vi "Icon_Adapt Format Cluster for Storage.vi"(8 "Error":errorcluster, 11 "Colors":T1={"Header"="", "Format"={"Color"={"Body txt"=255, "Body Back"=12632256, "Frame"=0, "Header txt"=32768, "Header Back"=16744703, "type"=enum."2 Color"}, "Icon Sizing"={"Rule"=enum."Static", "Header"=TRUE, "Rows"=5, "Width"=32, "Position"=enum."MID-CTR"}}} {"Format"."Icon Sizing"."Rows" min=1 max=5 step=1; "Format"."Icon Sizing"."Width" min=7 max=32 step=1}) -> (0 "Error Out":errorcluster, 3 "Colors Out":T1={"Header"="", "Format"={"Color"={"Body txt"=255, "Body Back"=12632256, "Frame"=0, "Header txt"=32768, "Header Back"=16744703, "type"=enum."2 Color"}, "Icon Sizing"={"Rule"=enum."Static", "Header"=TRUE, "Rows"=5, "Width"=32, "Position"=enum."MID-CTR"}}} {"Format"."Icon Sizing"."Rows" min=1 max=5 step=1; "Format"."Icon Sizing"."Width" min=7 max=32 step=1})   [LabVIEW 2009]
uses:
  Controls/Cluster/Cluster_Format Storage.ctl
  Controls/String_Picture/STRING_Line Display.ctl
  Controls/Cluster/Cluster_Icon Format.ctl
  Controls/Cluster/Cluster_Icon Color Set.ctl
  Controls/Enum/ENUM_Frame Template Select.ctl
  Controls/Cluster/Cluster_Sizing Data.ctl
  Controls/Enum/ENUM_Icon Sizing.ctl
  Controls/Enum/RBENUM_Icon Position.ctl
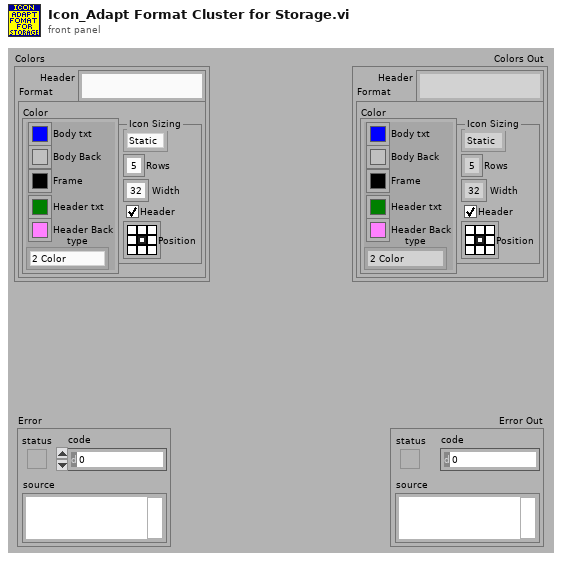
[diagram p1: front panel]
types:
  T1 = typedef "Cluster_Format Storage.ctl" = cluster{"Header":T2, "Format":T3}
  T2 = typedef "STRING_Line Display.ctl" = string
  T3 = typedef "Cluster_Icon Format.ctl" = cluster{"Color":T4, "Icon Sizing":T6}
  T4 = typedef "Cluster_Icon Color Set.ctl" = cluster{"Body txt":u32, "Body Back":u32, "Frame":u32, "Header txt":u32, "Header Back":u32, "type":T5}
  T5 = typedef "ENUM_Frame Template Select.ctl" = enum16{"2 Color", "5 Color"}
  T6 = typedef "Cluster_Sizing Data.ctl" = cluster{"Rule":T7, "Header":bool, "Rows":u32, "Width":u32, "Position":T8}
  T7 = typedef "ENUM_Icon Sizing.ctl" = enum16{"Static", "Auto"}
  T8 = typedef "RBENUM_Icon Position.ctl" = enum32{"LFT-TOP", "MID-TOP", "RGT-TOP", "LFT-CTR", "MID-CTR", "RGT-CTR", "LFT-BOT", "MID-BOT", "RGT-BOT"}
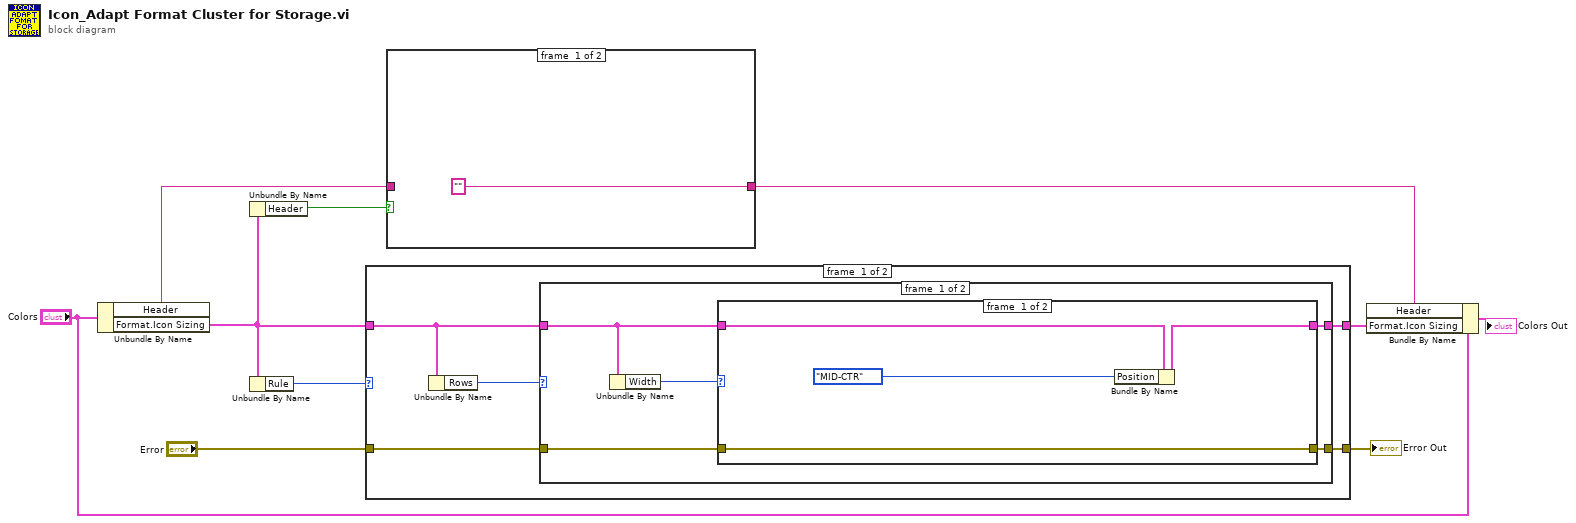
[diagram p0: block diagram]
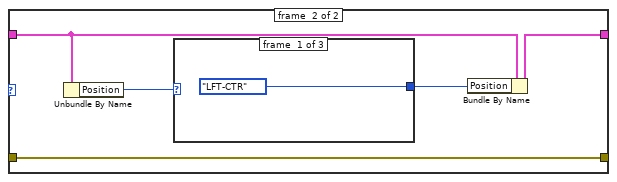
[diagram p3: hidden frame]
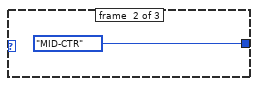
[diagram p4: hidden frame]
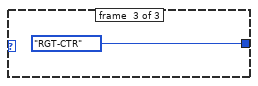
[diagram p5: hidden frame]
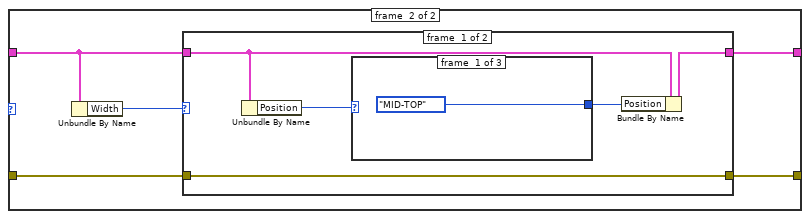
[diagram p6: hidden frame]
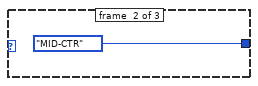
[diagram p7: hidden frame]
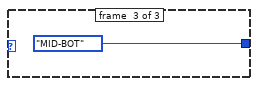
[diagram p8: hidden frame]
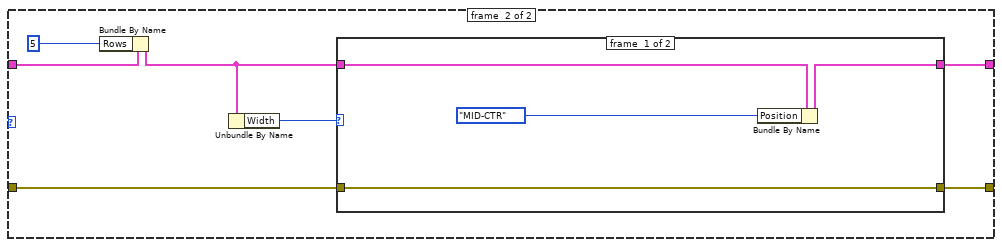
[diagram p10: hidden frame]
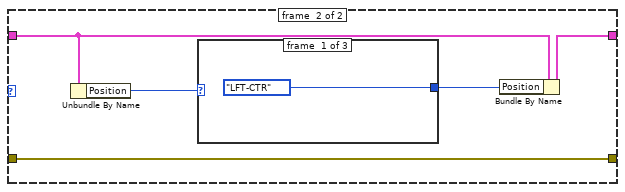
[diagram p11: hidden frame]
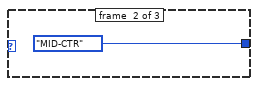
[diagram p12: hidden frame]
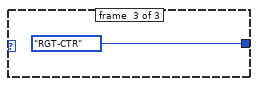
[diagram p13: hidden frame]
diagram:
  n1 = Unbundle By Name("Colors") -> ("Header"=w2:T2, "Format.Icon Sizing"=w4:T6)
  n2 = Unbundle By Name(w4) -> ("Header"=w3:bool)
  n3 = Unbundle By Name(w4) -> ("Rule"=w8:T7)
  n4 = case shown="\"Static\"" w8 {
    tunnel: [w13 w53] -> w10
    tunnel: "Error" -> [w14 w54]
    tunnel: w4 -> [w12 w50]
    tunnel: [w11 w52] -> w6
    frame #0 {
      n5 = Unbundle By Name(w12) -> ("Rows"=w15:u32)
      n6 = case shown="5.." w15 {
        tunnel: w14 -> [w16 w33]
        tunnel: [w17 w34] -> w13
        tunnel: w12 -> [w19 w36]
        tunnel: [w20 w37] -> w11
        frame #0 {
          n7 = Unbundle By Name(w19) -> ("Width"=w18:u32)
          n8 = case shown="..31" w18 {
            tunnel: [w22 w28] -> w20
            tunnel: w19 -> [w23 w27]
            tunnel: [w24 w29] -> w17
            tunnel: w16 -> [w24 w29]
            frame #0 {
              n9 = Bundle By Name(cluster=w23, "Position"=RBENUM_Icon_Position."MID-CTR" ("Icon Sizing.Position")) -> (w22:T6)
            }
            frame #1 {
              n10 = Unbundle By Name(w27) -> ("Position"=w26:T8)
              n11 = case shown="\"LFT-TOP\", \"LFT-CTR\", \"LFT-BOT\"" w26 {
                tunnel: [RBENUM_Icon_Position."LFT-CTR" ("Icon Sizing.Position") RBENUM_Icon_Position."MID-CTR" ("Icon Sizing.Position") RBENUM_Icon_Position."RGT-CTR" ("Icon Sizing.Position")] -> w25
                frame #0 {
                }
                frame #1 {
                }
                frame #2 {
                }
              }
              n12 = Bundle By Name(cluster=w27, "Position"=w25) -> (w28:T6)
            }
          }
        }
        frame #1 {
          n13 = Unbundle By Name(w36) -> ("Width"=w35:u32)
          n14 = case shown="32.." w35 {
            tunnel: [w41 w46] -> w37
            tunnel: w36 -> [w40 w46]
            tunnel: [w42 w47] -> w34
            tunnel: w33 -> [w42 w47]
            frame #0 {
              n15 = Unbundle By Name(w40) -> ("Position"=w39:T8)
              n16 = case shown="\"LFT-BOT\"..\"RGT-BOT\"" w39 {
                tunnel: [RBENUM_Icon_Position."MID-TOP" ("Icon Sizing.Position") RBENUM_Icon_Position."MID-CTR" ("Icon Sizing.Position") RBENUM_Icon_Position."MID-BOT" ("Icon Sizing.Position")] -> w38
                frame #0 {
                }
                frame #1 {
                }
                frame #2 {
                }
              }
              n17 = Bundle By Name(cluster=w40, "Position"=w38) -> (w41:T6)
            }
            frame #1 {
            }
          }
        }
      }
    }
    frame #1 {
      n18 = Bundle By Name(cluster=w50, "Rows"=u32 5 ("Icon Sizing.Rows")) -> (w49:T6)
      n19 = Unbundle By Name(w49) -> ("Width"=w51:u32)
      n20 = case shown="..31" w51 {
        tunnel: [w56 w62] -> w52
        tunnel: w49 -> [w57 w61]
        tunnel: [w58 w63] -> w53
        tunnel: w54 -> [w58 w63]
        frame #0 {
          n21 = Bundle By Name(cluster=w57, "Position"=RBENUM_Icon_Position."MID-CTR" ("Icon Sizing.Position")) -> (w56:T6)
        }
        frame #1 {
          n22 = Unbundle By Name(w61) -> ("Position"=w60:T8)
          n23 = case shown="\"LFT-TOP\", \"LFT-CTR\", \"LFT-BOT\"" w60 {
            tunnel: [RBENUM_Icon_Position."LFT-CTR" ("Icon Sizing.Position") RBENUM_Icon_Position."MID-CTR" ("Icon Sizing.Position") RBENUM_Icon_Position."RGT-CTR" ("Icon Sizing.Position")] -> w59
            frame #0 {
            }
            frame #1 {
            }
            frame #2 {
            }
          }
          n24 = Bundle By Name(cluster=w61, "Position"=w59) -> (w62:T6)
        }
      }
    }
  }
  "Error Out" <- w10
  n25 = case shown="True" w3 {
    tunnel: w2 -> [_ w68]
    tunnel: [T2 "" ("Header") w68] -> w1
    frame #0 {
    }
    frame #1 {
    }
  }
  n26 = Bundle By Name(cluster="Colors", "Header"=w1, "Format.Icon Sizing"=w6) -> (→"Colors Out":T1)
